vi "DAQmxTaskContainerUpdate-Com-Exec.vi"(8 "error in (no error)":errorcluster, 9 "data":variant, 10 "DAQmx Tasks":refnum<vi>, 11 "DAQmxTaskContainer in":refnum<class "DAQmxTaskContainer.lvclass">) -> (0 "error out":errorcluster, 3 "DAQmxTaskContainer out":refnum<class "DAQmxTaskContainer.lvclass">)   [LabVIEW 2015, in "DAQmxTaskContainer.lvclass"]
uses:
  DAQmxTaskContainer.lvclass
  GeneralFunctionality/GeneralFunctionality.lvclass/GeneralFunctionality.ctl
  Config/Config.lvclass/Config.ctl
  Config/Config.lvclass
  DAQmxTask.lvclass
  GeneralFunctionality/GeneralFunctionality.lvclass
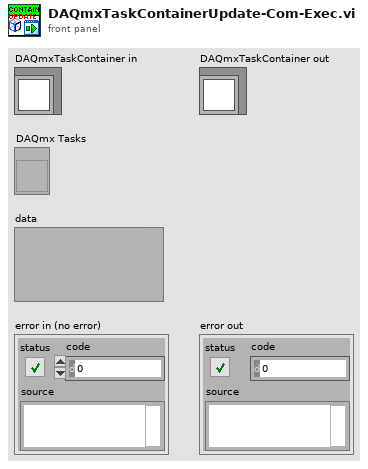
[diagram p1: front panel]
types:
  T1 = enum8{"Enabled", "Disabled", "Disabled and Grayed Out"}
  T2 = cluster{"name":string, "type of task":string, "Status":bool, "Value":string, "error":errorcluster}
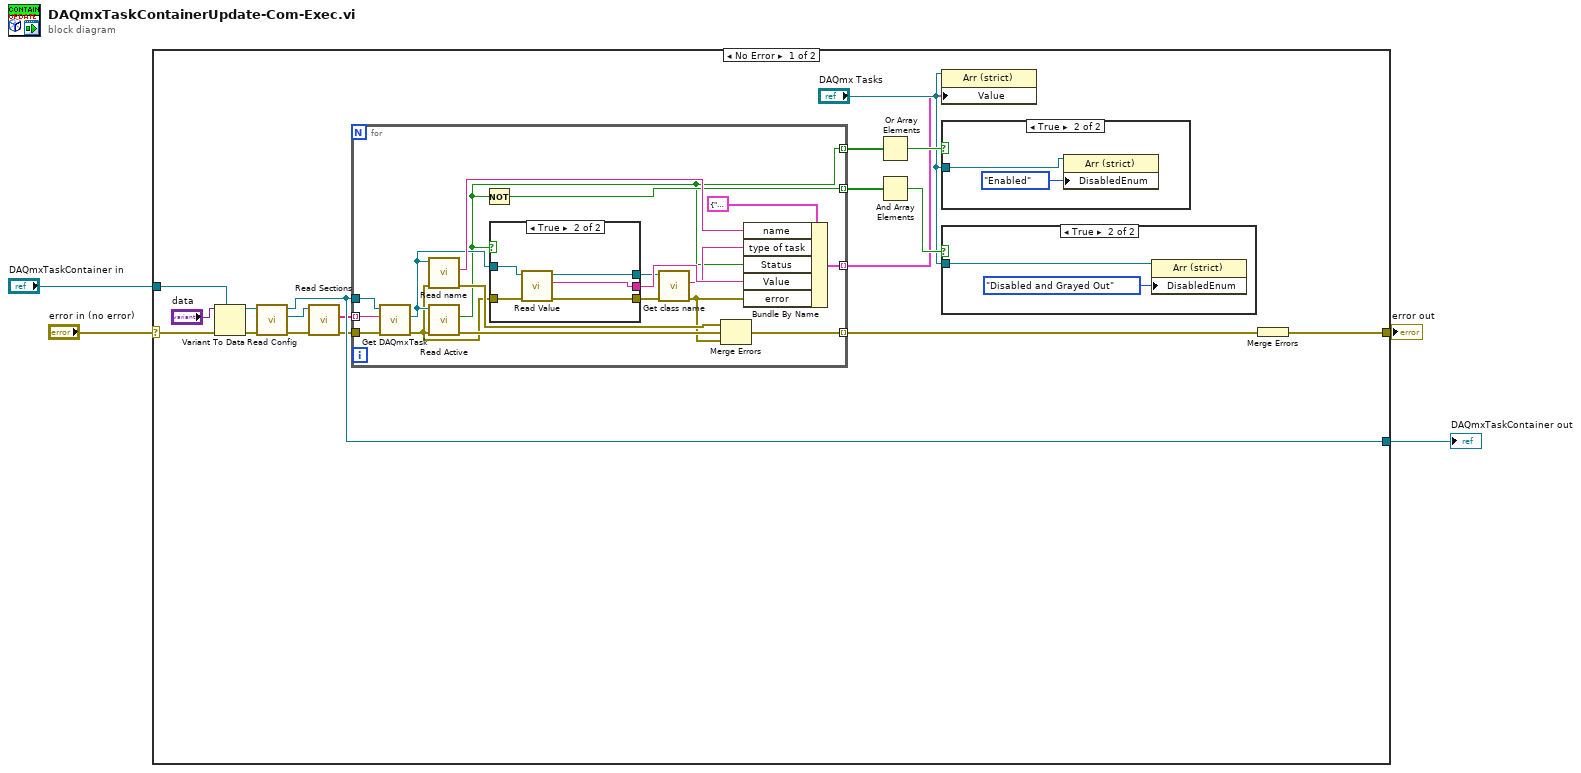
[diagram p0: block diagram]
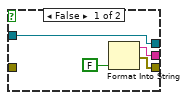
[diagram p4: hidden frame]
diagram:
  n1 = case shown="No Error" "error in (no error)" {
    selector: "error in (no error)" -> [w5 w55]
    tunnel: "DAQmxTaskContainer in" -> [w22 w54]
    tunnel: [w20 w55] -> w3
    tunnel: [w19 w54] -> w2
    frame No Error {
      n2 = Variant To Data(error in=w5, type=w22, Variant="data") -> (data=w9:refnum<class "DAQmxTaskContainer.lvclass">, error out=w8:errorcluster)
      n3 = call "Read Config.vi"("error in (no error)"=w8, "GeneralFunctionality en entrée"=w9) -> ("error out"=w18:errorcluster, "Config.lvclass"=w17:refnum<class "Config.lvclass">, "GeneralFunctionality en sortie"=w19:refnum<class "DAQmxTaskContainer.lvclass">)  [unwired: 7 in]
      n4 = call "Read Sections.vi"("error in (no error)"=w18, "Config in"=w17) -> ("error out"=w15:errorcluster, "Sections"=w16:string[])  [unwired: 7 in, 1 out]
      n5 = for {
        tunnel: w19 -> [w44]
        tunnel: w16 -> [w43] mode=indexing
        tunnel: w15 -> [w42]
        tunnel: [w36] -> w14 mode=indexing
        tunnel: [w35] -> w6 mode=indexing
        tunnel: [w28] -> w13 mode=indexing
        tunnel: [w27] -> w11 mode=indexing
        n6 = call "Get DAQmxTask.vi"("error in (no error)"=w42, "Task name"=w43, "DAQmxTaskContainer in"=w44) -> ("error out"=w33:errorcluster, "DAQmx Task"=w34:refnum<class "DAQmxTask.lvclass">)  [unwired: 6 in, 1 out]
        n7 = call "Read name.vi"("error in (no error)"=w33, "DAQmxTask in"=w34) -> ("error out"=w37:errorcluster, "name"=w40:string)  [unwired: 7 in, 1 out]
        n8 = call-dynamic "Read Active.vi"("error in (no error)"=w33, "DAQmxTask in"=w34) -> ("error out"=w38:errorcluster, "Active?"=w27:bool)  [unwired: 7 in, 1 out]
        n9 = Not(x=w27) -> (.not. x?=w28:bool)
        n10 = case shown="True" w27 {
          tunnel: [w47 w50] -> w39
          tunnel: [w48 w51] -> w31
          tunnel: w34 -> [w45 w53]
          tunnel: w33 -> [_ w52]
          tunnel: [w45 w49] -> w32
          frame False {
            n11 = Format Into String(FALSE ("input 1")) -> (resulting string=w47:string, error out=w48:errorcluster)  [unwired: 3 in]
          }
          frame True {
            n12 = call-dynamic "Read Value.vi"("error in (no error)"=w52, "DAQmxTask en entrée"=w53) -> ("error out"=w51:errorcluster, "Data string"=w50:string, "DAQmxTask en sortie"=w49:refnum<class "DAQmxTask.lvclass">)  [unwired: 6 in, 1 out]
          }
        }
        n13 = call "Get class name.vi"("error in (no error)"=w31, "DAQmxTask en entrée"=w32) -> ("error out"=w30:errorcluster, "Class name"=w29:string)  [unwired: 7 in, 1 out]
        n14 = Merge Errors(w37, w38, w30) -> (w36:errorcluster)
        n15 = Bundle By Name(cluster=T2 {"name"="", "type of task"="", "Status"=FALSE, "Value"="", "error"={"status"=FALSE, "code"=0, "source"=""}} ("Task"), "name"=w40, "type of task"=w29, "Status"=w27, "Value"=w39, "error"=w30) -> (w35:T2)
      }
      n16 = Or Array Elements(Boolean array=w11) -> (logical OR=w10:bool)
      n17 = And Array Elements(Boolean array=w13) -> (logical AND=w12:bool)
      n18 = property class="Arr (strict)"(reference="DAQmx Tasks", "Value"=w6) -> ()  [unwired: 1 in, 2 out]
      n19 = case shown="True" w10 {
        tunnel: "DAQmx Tasks" -> [_ w23]
        frame False {
        }
        frame True {
          n20 = property class="Arr (strict)"(reference=w23, "DisabledEnum"=T1."Enabled" ("Désactivé")) -> ()  [unwired: 1 in, 2 out]
        }
      }
      n21 = case shown="True" w12 {
        tunnel: "DAQmx Tasks" -> [_ w26]
        frame False {
        }
        frame True {
          n22 = property class="Arr (strict)"(reference=w26, "DisabledEnum"=T1."Disabled and Grayed Out" ("Désactivé")) -> ()  [unwired: 1 in, 2 out]
        }
      }
      n23 = Merge Errors(w14) -> (w20:errorcluster)
    }
    frame Error {
    }
  }
  "error out" <- w3
  "DAQmxTaskContainer out" <- w2
